vi "RemoveItem__slk_tc.vi"(0 "tree control in":refnum<class "TreeControl.lvclass">, 5 "input tag (current tag)":string, 11 "error in (no error)":errorcluster) -> (4 "tree control out":refnum<class "TreeControl.lvclass">, 15 "error out":errorcluster)   [LabVIEW 2020, in "TreeControl.lvclass"]
doc: "Deletes item from tree along with any children. Uses the current selection if there is no item input. If there is no item selected within the tree it deletes nothing. Returns error code 1136 if an invalid tag is passed in."
uses:
  Library/TreeControl.lvclass
  Library/TreeControl.lvclass/TreeControl.ctl
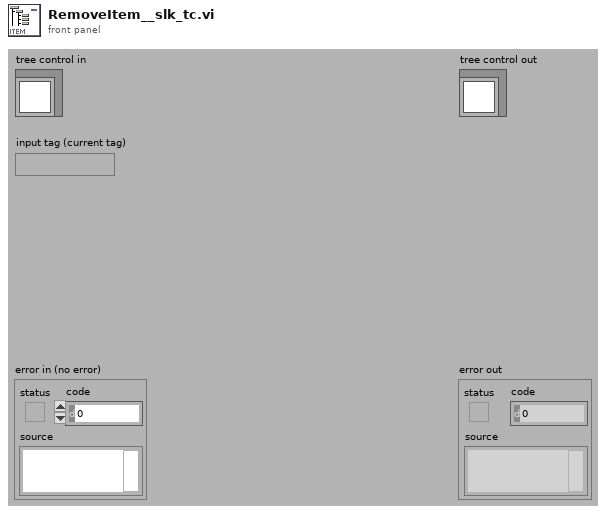
[diagram p1: front panel]
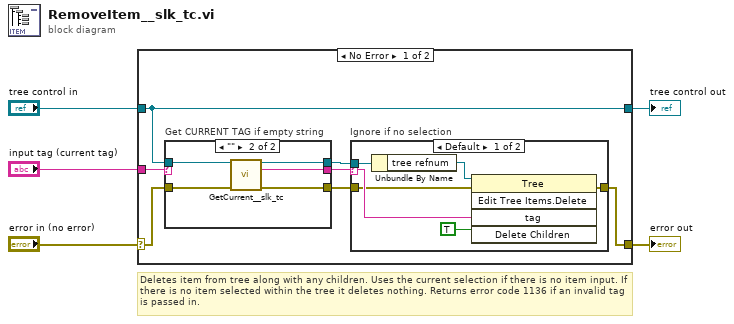
[diagram p0: block diagram]
diagram:
  # "Deletes item from tree along with any children. Uses the current selection if there is no item input. If there is no item selected within the tree it deletes nothing. Returns error code 1136 if an invalid tag is passed in."
  n1 = case shown="No Error" "error in (no error)" {
    selector: "error in (no error)" -> [w7 w29]
    tunnel: [w6 w29] -> w4
    tunnel: [w11 w28] -> w2
    tunnel: "tree control in" -> [w11 w28]
    tunnel: "input tag (current tag)" -> [w12 _]
    frame No Error {
      n2 = case "Get CURRENT TAG if empty string" shown="\"\"" w12 {
        selector: w12 -> [w22 _]
        tunnel: [w22 w27] -> w10
        tunnel: w11 -> [w20 w26]
        tunnel: w7 -> [w21 w25]
        tunnel: [w21 w24] -> w8
        tunnel: [w20 w23] -> w9
        frame Default {
        }
        frame "" {
          n3 = call "GetCurrent__slk_tc.vi"("tree control in"=w26, "error in (no error)"=w25) -> ("tree control out"=w23:refnum<class "TreeControl.lvclass">, "current tag"=w27:string, "error out"=w24:errorcluster)  [unwired: 1 in, 10 out]
        }
      }
      n4 = case "Ignore if no selection" shown="Default" w10 {
        selector: w10 -> [w16 _]
        tunnel: w9 -> [w18 _]
        tunnel: w8 -> [w15 w19]
        tunnel: [w13 w19] -> w6
        frame Default {
          n5 = Unbundle By Name(w18) -> ("tree refnum"=w17:refnum<vi>)
          n6 = invoke class="Tree" method="Edit Tree Items.Delete"(reference=w17, error in=w15, "tag"=w16, "Delete Children"=TRUE ("Delete Children?")) -> (error out=w13:errorcluster)  [unwired: 1 in, 4 out]
        }
        frame "" {
        }
      }
    }
    frame Error {
    }
  }
  "error out" <- w4
  "tree control out" <- w2
